vi "piezoEtlGetPosFromFirstCount.vi"(0 "firstFrameCount":u32, 1 "hamamatsuFrameCounterReferences":refnum<data-value>[](array[refnum]), 2 "piezoEtlPositionsReferences":refnum<data-value>[](array[refnum]), 3 "piezoEtlDerivativesReferences":refnum<data-value>[](array[refnum]), 4 "nFrames":u32) -> (5 "piezoEtlPositions":dbl[](array[numeric]), 6 "piezoEtlPositionsDerivatives":i16[](array[numeric]), 7 "success":bool)   [LabVIEW 2017]
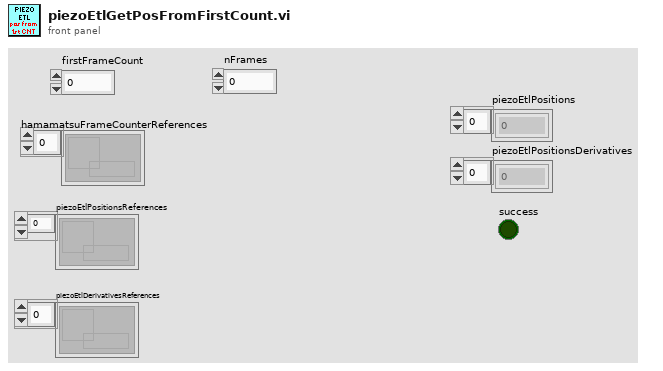
[diagram p1: front panel]
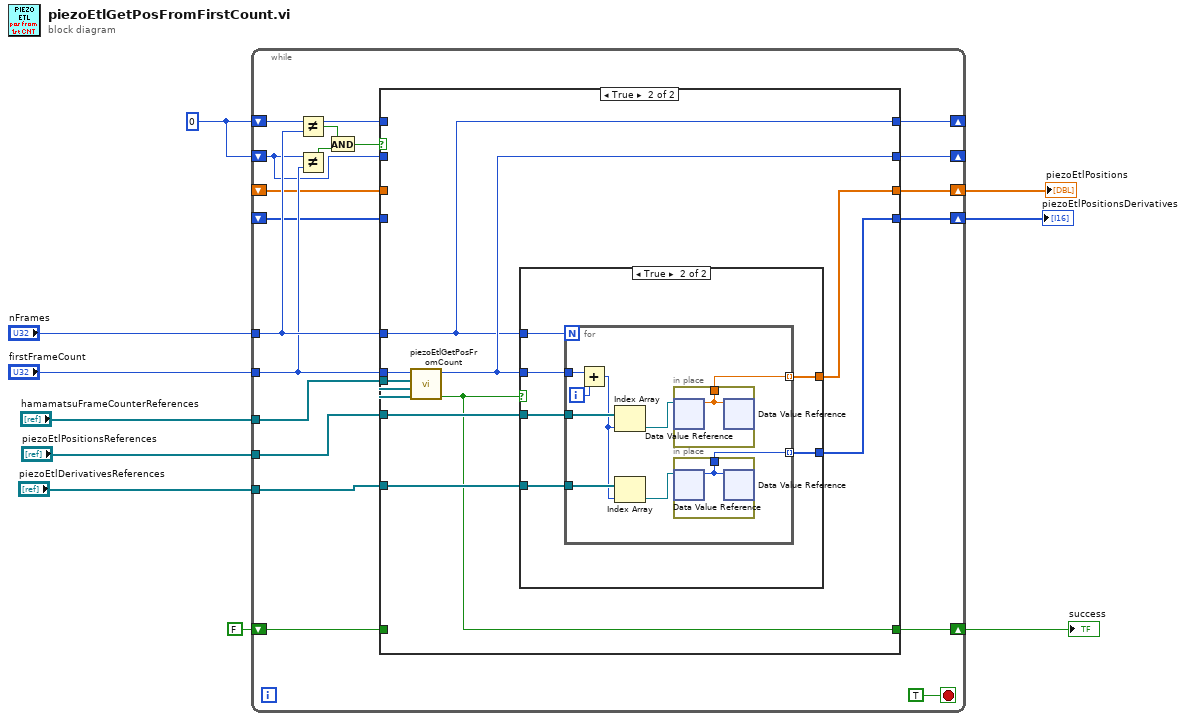
[diagram p0: block diagram]
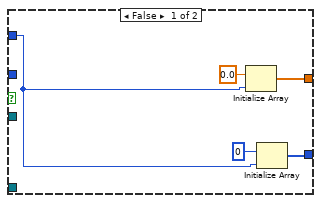
[diagram p3: hidden frame]
diagram:
  w2 = u32 0 ("nFrames")
  n1 = while {
    tunnel: "firstFrameCount" -> [w21]
    tunnel: "hamamatsuFrameCounterReferences" -> [w29]
    tunnel: "nFrames" -> [w22]
    tunnel: "piezoEtlPositionsReferences" -> [w28]
    tunnel: "piezoEtlDerivativesReferences" -> [w27]
    shift-right: [w15] -> _
    shift-left: w2 -> [w14]
    shift-right: [w23] -> _
    shift-left: w2 -> [w13]
    shift-right: [w26] -> w5
    shift-left: _ -> [w17]
    shift-right: [w25] -> w4
    shift-left: _ -> [w16]
    shift-right: [w24] -> w3
    shift-left: FALSE ("success") -> [w12]
    stop <- TRUE stop-if-true
    n2 = Not Equal?(x=w14, y=w22) -> (x != y?=w20:bool)
    n3 = Not Equal?(x=w13, y=w21) -> (x != y?=w19:bool)
    n4 = And(x=w20, y=w19) -> (x .and. y?=w18:bool)
    n5 = case shown="True" w18 {
      tunnel: w29 -> [_ w43]
      tunnel: w28 -> [_ w42]
      tunnel: w27 -> [_ w41]
      tunnel: [w34 w40] -> w26
      tunnel: [w33 w39] -> w25
      tunnel: [w30 w38] -> w24
      tunnel: [w32 w37] -> w23
      tunnel: w22 -> [_ w35]
      tunnel: w21 -> [_ w36]
      tunnel: w17 -> [w34 _]
      tunnel: w16 -> [w33 _]
      tunnel: [w31 w35] -> w15
      tunnel: w14 -> [w31 _]
      tunnel: w13 -> [w32 _]
      tunnel: w12 -> [w30 _]
      frame False {
      }
      frame True {
        n6 = call "piezoEtlGetPosFromCount.vi"("piezoEtlDerivativesReferences"=w41, "piezoEtlPositionsReferences"=w42, "hamamatsuFrameCounterReferences"=w43, "frameCount"=w36) -> ("success"=w38:bool, "bufferIndex"=w37:i32)  [unwired: 2 out]
        n7 = case shown="True" w38 {
          tunnel: w37 -> [_ w54]
          tunnel: w35 -> [w45 w53]
          tunnel: w42 -> [_ w52]
          tunnel: w41 -> [_ w51]
          tunnel: [w47 w50] -> w40
          tunnel: [w44 w49] -> w39
          frame False {
            n8 = Initialize Array(0.0 ("element"), w45) -> (w47:dbl[])
            n9 = Initialize Array(i16 0, w45) -> (w44:i16[])
          }
          frame True {
            n10 = for {
              N: w53 -> [_]
              tunnel: w54 -> [w57]
              tunnel: w52 -> [w63]
              tunnel: w51 -> [w59]
              tunnel: [w61] -> w50 mode=indexing
              tunnel: [w58] -> w49 mode=indexing
              i -> [w56]
              n11 = Add(x=w57, y=w56) -> (x+y=w55:i32)
              n12 = Index Array(array=w63, index=w55) -> (element=w62:refnum<data-value>)
              n13 = Index Array(array=w59, index=w55) -> (element=w60:refnum<data-value>)
              n14 = in-place {
                in-place-border: [w65] -> w61
                n15 = in-place-dvr #1(w62) -> (w65:dbl)  [unwired: 1 out]
                n16 = in-place-dvr #1(w65) -> ()  [unwired: 2 out]
              }
              n17 = in-place {
                in-place-border: [w64] -> w58
                n18 = in-place-dvr #2(w60) -> (w64:i16)  [unwired: 1 out]
                n19 = in-place-dvr #2(w64) -> ()  [unwired: 2 out]
              }
            }
          }
        }
      }
    }
  }
  "piezoEtlPositions" <- w5
  "piezoEtlPositionsDerivatives" <- w4
  "success" <- w3
